vi "ZLIB Delete Files From Archive__ogtk.vi"(8 "error in (no error)":errorcluster, 10 "files to delete":path[](array[path]), 11 "archive name (file dialog)":path) -> (0 "error out":errorcluster, 3 "archive name out":path)   [LabVIEW 2011]
doc: "This function accepts a zip archive file name and deletes the specified files from it. It does this by creating a temporary file and copying all files which must not be deleted into this file and when everything was successful, it replaces the original archive with the temporary copy.\nThe copying happens in raw mode which means that the files are not decompressed and compressed again and also that even password protected files are just copied over into the new archive without any problems, keeping their passwords."
uses:
  file/file.llb/Valid Path - Traditional__ogtk.vi
  ZLIB Open Zip Archive__ogtk.vi
  ZLIB Open Unzip Archive__ogtk.vi
panel:
  # "Please visit http://www.OpenG.org to learn about the\nOpen Source LabVIEW software movement.\n\nNOTICE -- YOU MUST LEAVE THIS NOTICE IN PLACE.  PER THE TERMS OF THE LICENSE BELOW, YOU MAY SUBLICENSE THIS SOFTWARE \nIN ANY WAY THAT DOES NOT CONFLICT WITH THIS LICENSE.\n\n### BSD License (http://www.opensource.org/licenses/bsd-license.php) Begin ###\n \nCopyright (C) 2004 Rolf Kalbermatter rolf.kalbermatter@citeng.com\n\nAll rights reserved.\n\nRedistribution and use in source and binary forms, with or without modification, are permitted provided that the following conditions are met:\n\n    * Redistributions of source code must retain the above copyright notice, this list of conditions and the following disclaimer.\n    * Redistributions in binary form must reproduce the above copyright notice, this list of conditions and the following disclaimer in the \n       documentation and/or other materials provided with the distribution.\n    * Neither the name of SciWare, James Kring, Inc., nor the names of its contributors may be used to endorse or promote products derived \n       from this software without specific prior written permission.\n\nTHIS SOFTWARE IS PROVIDED BY THE COPYRIGHT HOLDERS AND CONTRIBUTORS \"AS IS\" AND ANY EXPRESS OR IMPLIED WARRANTIES, \nINCLUDING, BUT NOT LIMITED TO, THE IMPLIED WARRANTIES OF MERCHANTABILITY AND FITNESS FOR A PARTICULAR PURPOSE ARE \nDISCLAIMED. IN NO EVENT SHALL THE COPYRIGHT OWNER OR CONTRIBUTORS BE LIABLE FOR ANY DIRECT, INDIRECT, INCIDENTAL,\n SPECIAL, EXEMPLARY, OR CONSEQUENTIAL DAMAGES (INCLUDING, BUT NOT LIMITED TO, PROCUREMENT OF SUBSTITUTE GOODS OR \nSERVICES; LOSS OF USE, DATA, OR PROFITS; OR BUSINESS INTERRUPTION) HOWEVER CAUSED AND ON ANY THEORY OF LIABILITY, \nWHETHER IN CONTRACT, STRICT LIABILITY, OR TORT (INCLUDING NEGLIGENCE OR OTHERWISE) ARISING IN ANY WAY OUT OF THE USE \nOF THIS SOFTWARE, EVEN IF ADVISED OF THE POSSIBILITY OF SUCH DAMAGE.\n\n### BSD License End ###"
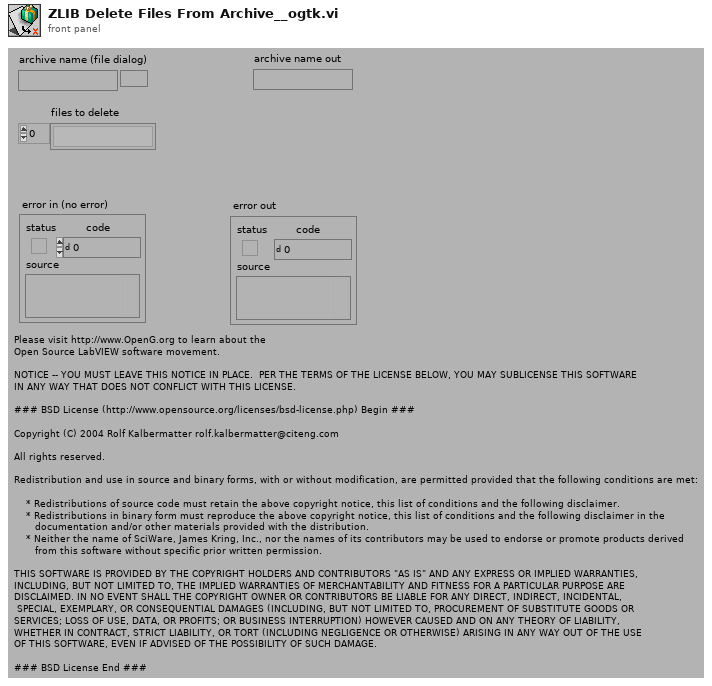
[diagram p1: front panel]
types:
  T1 = enum32{"existing file", "new file", "new or existing file", "existing dir", "new dir", "new or existing dir", "existing file (use LLBs)", "new file (use LLBs)", "new or existing file (use LLBs)", "new or existing file or directory (use LLBs)", "existing dir (use LLBs)", "new dir (use LLBs)", "new or existing dir (use LLBs)", "existing file or dir", "new file or dir", "new or existing file or dir", "existing file or dir (use LLBs)", "new file or dir (use LLBs)"}
  T2 = typedef "ZLIB Zip Handle__ogtk.ctl" = refnum<k1>
  T3 = typedef "ZLIB Unzip Handle__ogtk.ctl" = refnum<k1>
  T4 = typedef "ZLIB File Info__ogtk.ctl" = cluster{"version":u32, "version needed":u32, "encrypted":bool, "flag":u32, "compression":i32, "dos date":u32, "crc":u32, "compressed size":u32, "uncompressed size":u32, "extra info":string, "file comment":string, "disk num start":u32, "internal fa":u32, "external fa":u32, "file timestamp":u32}
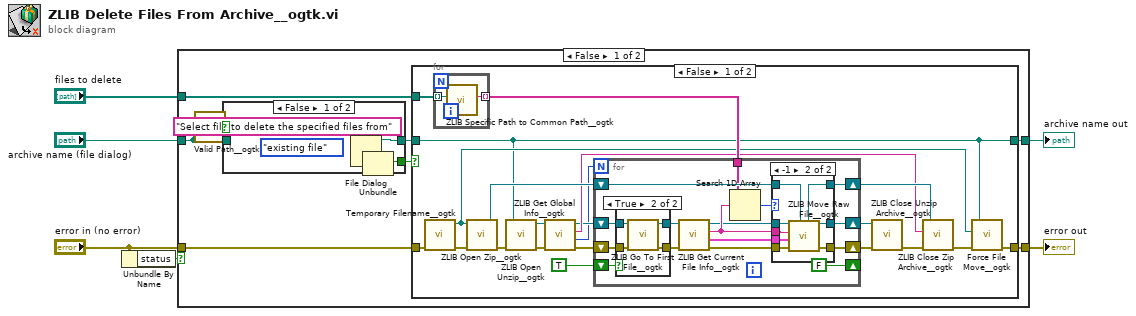
[diagram p0: block diagram]
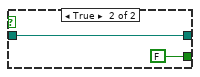
[diagram p2: hidden frame]
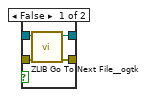
[diagram p3: hidden frame]
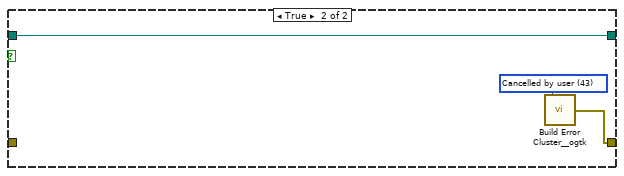
[diagram p5: hidden frame]
diagram:
  n1 = Unbundle By Name("error in (no error)") -> ("status"=w4:bool)
  n2 = case shown="False" w4 {
    tunnel: "archive name (file dialog)" -> [w12 w82]
    tunnel: "error in (no error)" -> [w10 w83]
    tunnel: [w9 w83] -> w3
    tunnel: [w8 w82] -> w2
    tunnel: "files to delete" -> [w7 _]
    frame False {
      n3 = call-poly "Valid Path__ogtk.vi"("path"=w12) -> ("valid"=w11:bool)
      n4 = case shown="False" w11 {
        tunnel: [w17 w20] -> w14
        tunnel: [w16 FALSE ("cancelled")] -> w13
        tunnel: w12 -> [_ w20]
        frame False {
          (unwired) T1."existing file" ("select mode (2)")
          n5 = File Dialog(7:"Select file to delete the specified files from" ("prompt")) -> (0:w15:errorcluster, 1:w16:bool, 3:w17:path)  [unwired: 6 in, 1 out]
          n6 = Unbundle(w15) -> ()  [unwired: 3 out]
        }
        frame True {
        }
      }
      n7 = case shown="False" w13 {
        tunnel: w14 -> [w28 w79]
        tunnel: [w32 w80] -> w9
        tunnel: w7 -> [w38 _]
        tunnel: w10 -> [w34 _]
        tunnel: [w28 w79] -> w8
        frame False {
          n8 = call "Temporary Filename__ogtk.vi"("error in (no error)"=w34) -> ("error out"=w31:errorcluster, "file in tmp dir"=w29:path)  [unwired: 5 in]
          n9 = for {
            tunnel: w38 -> [w43] mode=indexing
            tunnel: [w42] -> w37 mode=indexing
            n10 = call "ZLIB Specific Path to Common Path__ogtk.vi"("specific path"=w43) -> ("common path"=w42:string)  [unwired: 10 in]
          }
          n11 = call-poly "ZLIB Open Zip__ogtk.vi"("error in (no error)"=w31, "archive name"=w29) -> ("error out"=w30:errorcluster, "zip Refnum"=w40:T2)  [unwired: 3 in, 1 out]
          n12 = call-poly "ZLIB Open Unzip__ogtk.vi"("error in (no error)"=w30, "archive name"=w28) -> ("error out"=w27:errorcluster, "unzip Refnum"=w26:T3)  [unwired: 4 in]
          n13 = call "ZLIB Get Global Info__ogtk.vi"("error in (no error)"=w27, "unzip Refnum"=w26) -> ("error out"=w24:errorcluster, "nEntry"=w22:u32, "global comment"=w25:string, "unzip Refnum out"=w23:T3)  [unwired: 2 in]
          n14 = for {
            N: w22 -> [_]
            shift-right: [w59] -> w41
            shift-left: w23 -> [w52]
            shift-right: [w58] -> w36
            shift-left: w24 -> [w53]
            shift-right: [w57] -> w39
            shift-left: w40 -> [w56]
            tunnel: w37 -> [w55]
            shift-right: [FALSE] -> _
            shift-left: TRUE -> [w50]
            n15 = case shown="True" w50 {
              tunnel: w52 -> [w62 w67]
              tunnel: w53 -> [w63 w66]
              tunnel: [w61 w65] -> w51
              tunnel: [w60 w64] -> w49
              frame False {
                n16 = call "ZLIB Go To Next File__ogtk.vi"("error in (no error)"=w63, "unzip Refnum"=w62) -> ("error out"=w60:errorcluster, "unzip Refnum out"=w61:T3)  [unwired: 4 in]
              }
              frame True {
                n17 = call "ZLIB Go To First File__ogtk.vi"("error in (no error)"=w66, "unzip Refnum"=w67) -> ("error out"=w64:errorcluster, "unzip Refnum out"=w65:T3)  [unwired: 4 in]
              }
            }
            n18 = call "ZLIB Get Current File Info__ogtk.vi"("error in (no error)"=w49, "unzip Refnum"=w51) -> ("error out"=w46:errorcluster, "file info"=w45:T4, "name"=w48:string, "unzip Refnum out"=w47:T3)  [unwired: 6 in]
            n19 = Search 1D Array(1D array=w55, element=w48) -> (index of element=w54:i32)  [unwired: 1 in]
            n20 = case shown="-1" w54 {
              tunnel: [w70 w73] -> w59
              tunnel: [w68 w74] -> w58
              tunnel: [w69 w72] -> w57
              tunnel: w56 -> [w69 w71]
              tunnel: w47 -> [w70 w78]
              tunnel: w46 -> [w68 w75]
              tunnel: w48 -> [_ w77]
              tunnel: w45 -> [_ w76]
              frame 0, Default {
              }
              frame -1 {
                n21 = call "ZLIB Move Raw File__ogtk.vi"("zip Refnum"=w71, "error in (no error)"=w75, "file info"=w76, "name"=w77, "unzip Refnum"=w78) -> ("error out"=w74:errorcluster, "unzip Refnum out"=w73:T3, "zip Refnum out"=w72:T2)  [unwired: 4 in]
              }
            }
          }
          n22 = call "ZLIB Close Unzip Archive__ogtk.vi"("error in (no error)"=w36, "unzip Refnum"=w41) -> ("error out"=w35:errorcluster)  [unwired: 5 in]
          n23 = call "ZLIB Close Zip Archive__ogtk.vi"("error in (no error)"=w35, "global comment (use original comment for existing files)"=w25, "zip Refnum"=w39) -> ("error out"=w33:errorcluster)  [unwired: 3 in, 1 out]
          n24 = call "Force File Move__ogtk.vi"("error in (no error)"=w33, "source"=w29, "target"=w28) -> ("error out"=w32:errorcluster)  [unwired: 3 in, 1 out]
        }
        frame True {
          w81 = 43 items=["No error", "Argument error", "Memory is full", "Out of zone", "End of file", "File already open", "Generic file I/O error", "File not found", "File permission error", "Disk is full", "Duplicate path", "Too many files open", "System feature not enabled", "Resource file not found", "Cannot add resource", "Resource not found", "Image not found", "Image memory error", "Pen does not exist", "Config type invalid", "Config token not found", "Config parse error", "Config memory error", "Bad external code format", "Bad external code offset", "External code not present", "Null window", "Destroy window error", "Null menu", "Print aborted", "Bad print record", "Print driver error", "Windows error during printing", "Memory error during printing", "Print dialog error", "Generic print error", "Invalid device refnum", "Device not found", "Device parameter error", "Device unit error", "Cannot open device", "Device call aborted", "Generic error", "Cancelled by user", "Object ID too low", "Object ID too high", "Object not in heap", "Unknown heap", "Unknown object (invalid DefProc)", "Unknown object (DefProc not in table)", "Message out of range", "Invalid (null) method", "Unknown message", "Manager call not supported", "Bad address", "Network operation in progress", "Network operation timed out", "Connection is busy", "Network attribute not supported", "Network error", "Address in use", "System out of memory", "Connection aborted", "Connection refused", "Not connected", "Already connected", "Connection closed", "Initialization error (interapplication manager)", "Bad occurrence", "Wait on unbound occurrence handler", "Occurrence queue overflow", "Datalog type conflict", "Unused", "Unrecognized type (interapplication manager)", "Memory corrupt", "Failed to make temporary DLL", "Old CIN version", "Drag socket not found", "Failed to load drop-object", "Failed to register OLE object", "Failed to release OLE object", "Format specifier type mismatch", "Unknown format specifier", "Too few format specifiers", "Too many format specifiers", "Scan failed", "Newer CIN version", "Error converting to variant", "Runtime menu error", "Password tampered", "Variant attribute not found", "Incompatible variant data type", "Event data is not available", "Event Store is not present", "Occurrence is not found", "Event Queue is not created", "Event info is not available", "Refnum passed is NULL", "Error retrieving Class GUID", "Error retrieving CoClass GUID", "Error retrieving TypeLib GUID.", "Bad built application magic bytes.", "Specific driver is different from the specific driver associated with the Logical Name.", "There is no session opened to the class driver.", "Max Error", "MAX - Error with config objects", "MAX - Error loading configuration", "MAX - Group not supported"]
          n25 = call "Build Error Cluster__ogtk.vi"("code"=w81) -> ("error out"=w80:errorcluster)  [unwired: 1 in]
        }
      }
    }
    frame True {
    }
  }
  "error out" <- w3
  "archive name out" <- w2
